vi "MH_AllocateCntRateBuffer.vi"(11 "NumChan":i32) -> (3 "Buffer":i32[](array[numeric]))   [LabVIEW 2010]
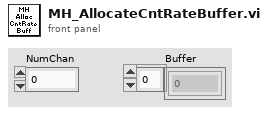
[diagram p1: front panel]
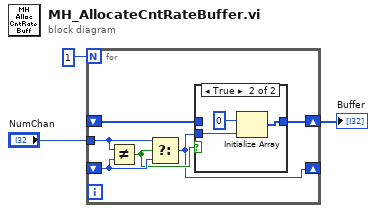
[diagram p0: block diagram]
diagram:
  n1 = for {
    N: 1 -> [_]
    shift-right: [w6] -> _
    shift-left: _ -> [w8]
    tunnel: "NumChan" -> [w9]
    shift-right: [w5] -> w3
    shift-left: _ -> [w4]
    n2 = Not Equal?(x=w9, y=w8) -> (x != y?=w7:bool)
    n3 = Select(t=w9, s=w7, f=w8) -> (s? t:f=w6:i32)
    n4 = case shown="True" w7 {
      tunnel: w6 -> [_ w13]
      tunnel: [w10 w11] -> w5
      tunnel: w4 -> [w10 _]
      frame False {
      }
      frame True {
        n5 = Initialize Array(0, w13) -> (w11:i32[])
      }
    }
  }
  "Buffer" <- w3
